vi "main.vi"() -> ()   [LabVIEW 2017]
uses:
  <vilib>/DAQmx/create/channels.llb/DAQmx Create Channel (AO-Voltage-Basic).vi
  <vilib>/DAQmx/configure/timing.llb/DAQmx Timing (Use Waveform).vi
panel:
  in  "physical channels":tag
  in  "Filename":path=path "test.tdms"
  out "Thermocouple":dynamicdata(graph)
  out "Thermocouples \n(Celsius)":dbl[](array[numeric])
  in  "stop 2":bool
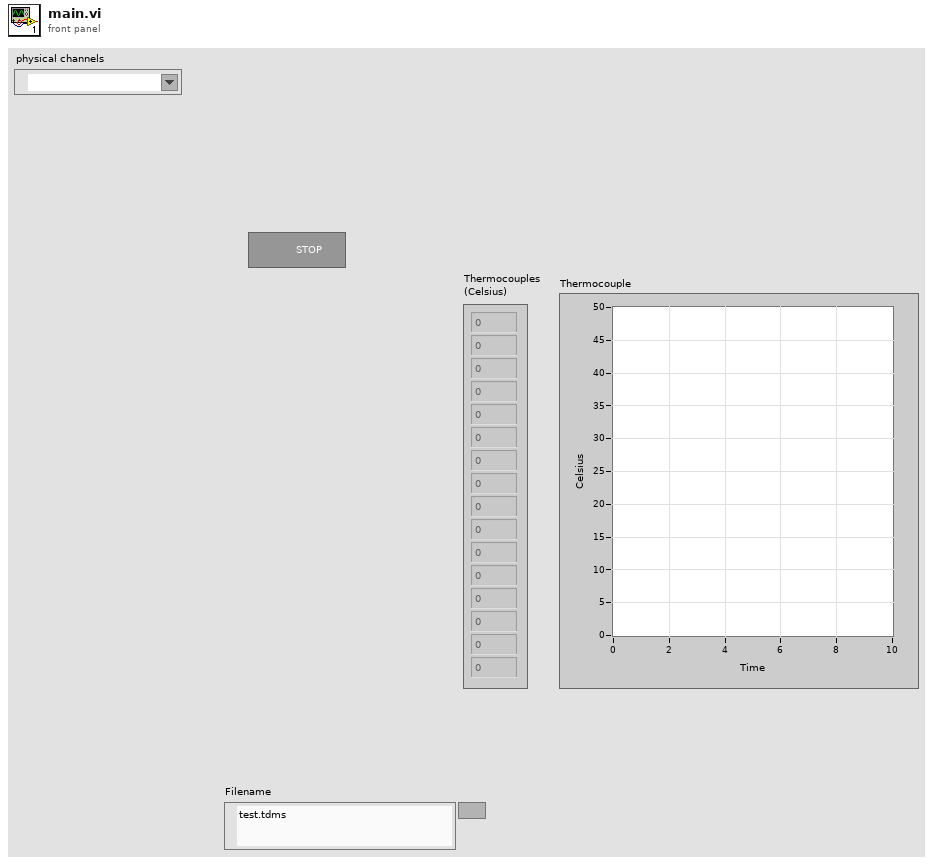
[diagram p1: front panel]
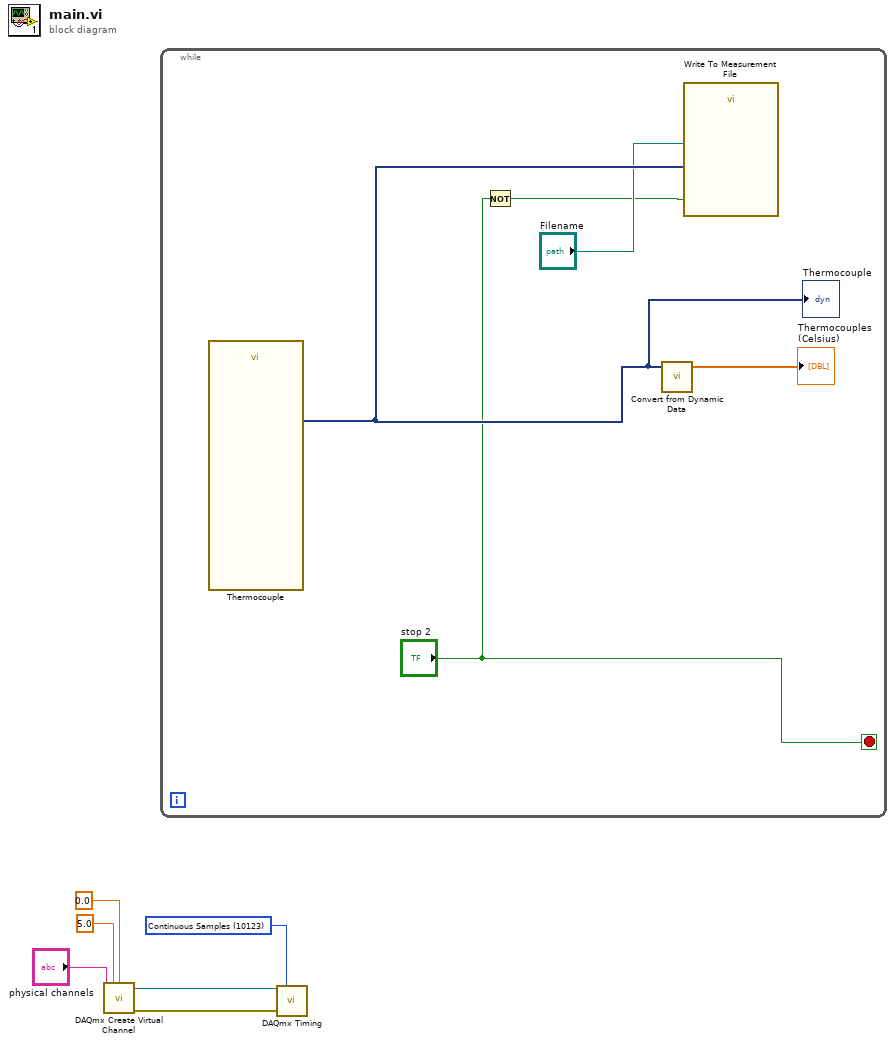
[diagram p0: block diagram]
diagram:
  w5 = 10123 items=["Finite Samples"=10178, "Continuous Samples"=10123, "Hardware Timed Single Point"=12522] ("sample mode")
  n1 = call-poly <vilib>:"DAQmx Create Virtual Channel.vi"("maximum value"=5.0, "minimum value"=0.0, "physical channels"="physical channels") -> ("task out"=w3:refnum<k21>, "error out"=w4:errorcluster)  [unwired: 11 in]
  n2 = while {
    stop <- "stop 2" stop-if-true
    n3 = call "Thermocouple"() -> ("data"=w10:dynamicdata)  [unwired: 16 in, 3 out]
    "Thermocouple" <- w10
    n4 = Not(x="stop 2") -> (.not. x?=w7:bool)
    n5 = call "Convert from Dynamic Data"("Dynamic Data Type"=w10) -> ("Array"=→"Thermocouples \n(Celsius)":dbl[])  [unwired: 3 in]
    n6 = call "Write To Measurement File"("Signals"=w10, "Flush? (T)"=w7, "Filename"="Filename") -> ()  [unwired: 14 in, 3 out]
  }
  n7 = call-poly <vilib>:"DAQmx Timing.vi"("task/channels in"=w3, "sample mode"=w5, "error in"=w4) -> ()  [unwired: 11 in, 2 out]
